vi "[RT]DisplayMain.vi"() -> (10 "Prozent schon gekocht":dbl(slide) scale=0.0..100.0, 11 "Anzahl der Tassen Kaffee":dbl)   [LabVIEW 2018]
doc: "The myRIO Project template acquires acceleration data from the onboard accelerometer and displays the changes of acceleration values in a waveform chart."
uses:
  <vilib>/Instr/_visa.llb/VISA Configure Serial Port (Instr).vi
  RT/[GlobVar]SensorState.vi
panel:
  out "error out":errorcluster
  in  "Stop":bool
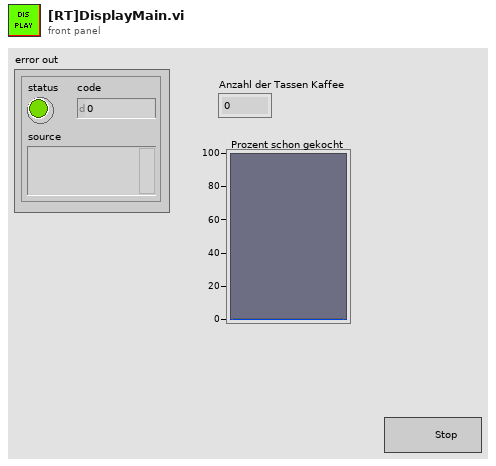
[diagram p1: front panel]
types:
  T1 = typedef "ControllerState.ctl" = enum16{"Idle", "Vorheizen", "Brühen", "Emergency-Stop"}
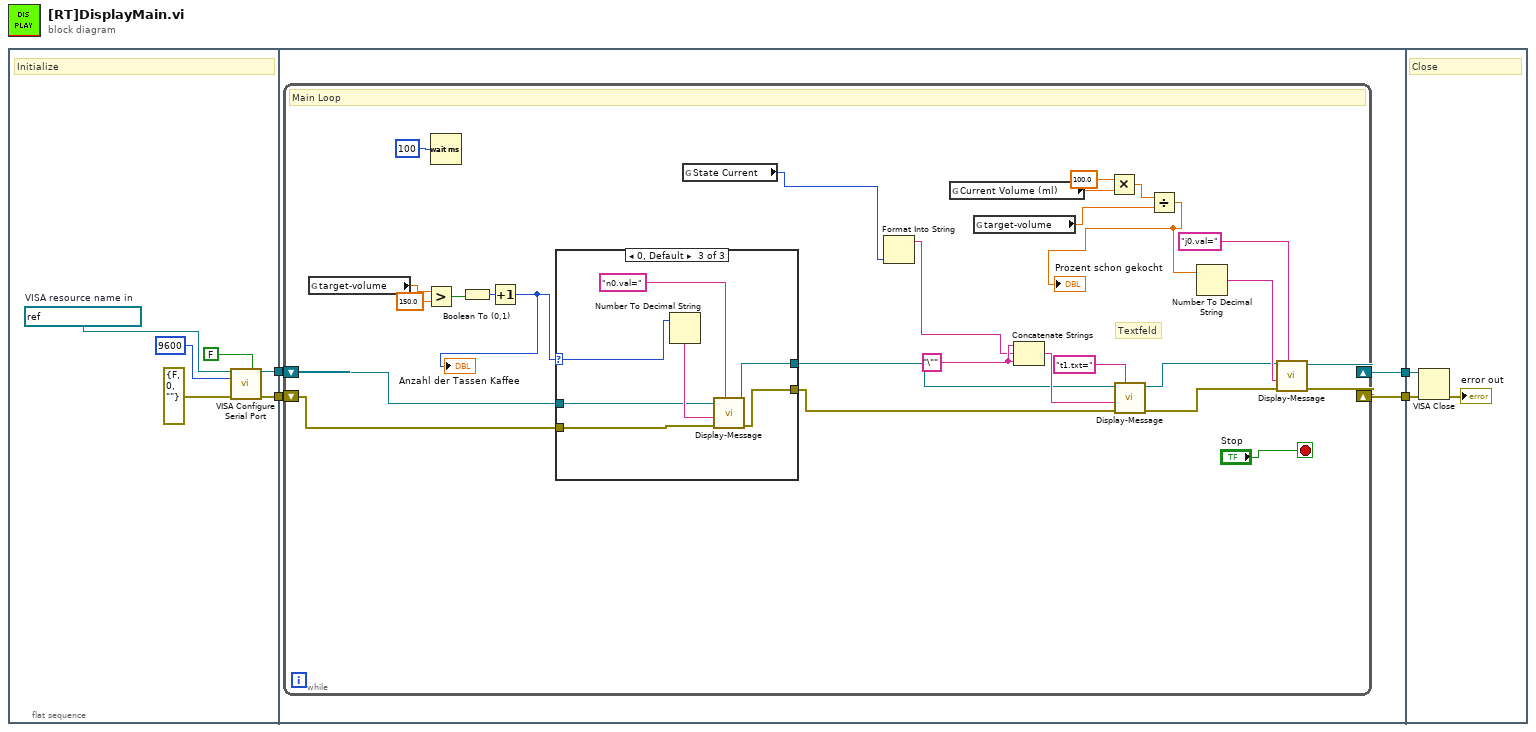
[diagram p0: block diagram]
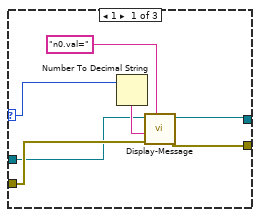
[diagram p2: hidden frame]
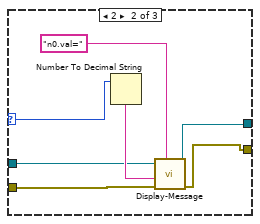
[diagram p3: hidden frame]
diagram:
  n1 = flat-sequence {
    tunnel: [w6] -> w4
    tunnel: [w7] -> w2
    tunnel: w4 -> [w14]
    tunnel: [w13] -> w3
    tunnel: w2 -> [w12]
    tunnel: [w11] -> w1
    tunnel: w3 -> [w64]
    tunnel: w1 -> [w65]
    frame #0 {
      w8 = refnum<visa-resource-name> "ASRL1::INSTR"  # VISA resource name in
      # "Initialize"
      n2 = call-poly "VISA Configure Serial Port"("VISA resource name"=w8, "Enable Termination\nChar (T)"=FALSE ("Enable Termination\nChar (T)"), "baud rate (9600)"=u32 9600, "error in (no error)"=errorcluster {"status"=FALSE, "code"=0, "source"=""}) -> ("VISA resource name out"=w7:refnum<visa-resource-name>, "error out"=w6:errorcluster)  [unwired: 10 in]
    }
    frame #1 {
      n3 = while {
        shift-right: [w35] -> w13
        shift-left: w14 -> [w37]
        shift-right: [w34] -> w11
        shift-left: w12 -> [w36]
        stop <- "Stop" stop-if-true
        w33 = "\""
        # "Textfeld"
        # "Main Loop"
        n4 = global read "[GlobVar]SensorState.vi" "target-volume"() -> (w21:dbl)
        n5 = Greater?(x=w21, y=150.0) -> (0:w19:bool)
        n6 = Wait (ms)(milliseconds to wait=u32 100) -> ()  [unwired: 1 out]
        n7 = Boolean To (0,1)(Boolean=w19) -> (0, 1=w18:i16)
        n8 = Increment(x=w18) -> (x+1=w17:i16)
        "Anzahl der Tassen Kaffee" <- w17
        n9 = case shown="0, Default" w17 {
          selector: w17 -> [w42 w49 w56]
          tunnel: w37 -> [w44 w51 w60]
          tunnel: w36 -> [w43 w50 w59]
          tunnel: [w45 w53 w58] -> w29
          tunnel: [w46 w52 w57] -> w30
          frame 1 {
            n10 = Number To Decimal String(number=w42) -> (decimal integer string=w48:string)  [unwired: 1 in]
            n11 = call "Display-Message.vi"("Element"="n0.val=", "error in (no error)"=w44, "Message"=w48, "VISA Refnum in"=w43) -> ("error out"=w45:errorcluster, "VISA Refnum out"=w46:refnum<visa-resource-name>)  [unwired: 6 in]
          }
          frame 2 {
            n12 = Number To Decimal String(number=w49) -> (decimal integer string=w55:string)  [unwired: 1 in]
            n13 = call "Display-Message.vi"("Element"="n0.val=", "error in (no error)"=w51, "Message"=w55, "VISA Refnum in"=w50) -> ("error out"=w53:errorcluster, "VISA Refnum out"=w52:refnum<visa-resource-name>)  [unwired: 6 in]
          }
          frame 0, Default {
            n14 = Number To Decimal String(number=w56) -> (decimal integer string=w62:string)  [unwired: 1 in]
            n15 = call "Display-Message.vi"("Element"="n0.val=", "error in (no error)"=w60, "Message"=w62, "VISA Refnum in"=w59) -> ("error out"=w58:errorcluster, "VISA Refnum out"=w57:refnum<visa-resource-name>)  [unwired: 6 in]
          }
        }
        n16 = global read "[GlobVar]SensorState.vi" "State Current"() -> (w15:T1)
        n17 = Format Into String(w15) -> (resulting string=w26:string)  [unwired: 3 in, 1 out]
        n18 = global read "[GlobVar]SensorState.vi" "Current Volume (ml)"() -> (w25:dbl)
        n19 = global read "[GlobVar]SensorState.vi" "target-volume"() -> (w22:dbl)
        n20 = Concatenate Strings(w33, w26, w33) -> (w31:string)
        n21 = Multiply(x=100.0, y=w25) -> (x*y=w23:dbl)
        n22 = call "Display-Message.vi"("Element"="t1.txt=", "error in (no error)"=w29, "Message"=w31, "VISA Refnum in"=w30) -> ("error out"=w27:errorcluster, "VISA Refnum out"=w28:refnum<visa-resource-name>)  [unwired: 6 in]
        n23 = Divide(x=w23, y=w22) -> (x/y=w16:dbl)
        "Prozent schon gekocht" <- w16
        n24 = Number To Decimal String(number=w16) -> (decimal integer string=w39:string)  [unwired: 1 in]
        n25 = call "Display-Message.vi"("Element"="j0.val=", "error in (no error)"=w27, "Message"=w39, "VISA Refnum in"=w28) -> ("error out"=w35:errorcluster, "VISA Refnum out"=w34:refnum<visa-resource-name>)  [unwired: 6 in]
      }
    }
    frame #2 {
      # "Close"
      n26 = VISA Close(VISA resource name=w65, error in (no error)=w64) -> (error out=→"error out":errorcluster)
    }
  }
